vi "fpga_96ch-Main_dead_pixels.vi"   [LabVIEW 2011]
uses:
  <vilib>/Platform/TimedLoop/XDataNode/timing_clust.ctl
  <vilib>/Platform/TimedLoop/XDataNode/nitl_modes.ctl
  <vilib>/Platform/TimedLoop/XDataNode/wakeup.ctl
  <vilib>/Platform/TimedLoop/XDataNode/XDataNode.xnode
  <vilib>/Platform/TimedLoop/XDataNode/XDNodeRunTimeDep.lvlib
types:
  T1 = typedef "XDNodeRunTimeDep.lvlib/timing_clust.ctl" = cluster{"Expected End [f-1]":u64, "Actual End [f-1]":u64, "Finished Late? [f-1]":bool, "Expected End [i-1]":u64, "Actual End [i-1]":u64, "Finished Late? [i-1]":bool, "Expected Start [i]":u64, "Actual Start [i]":u64, "Expected Start [f]":u64, "Actual Start [f]":u64, "Source Name":string, "Structure Name":string, "Period":i64, "Deadline":i64, "Offset":i64, "Start":i64, "Priority":i32, "Timeout":i32, "Mode":T2, "Wakeup Reason":T3, "Error":errorcluster, "Source Type":string, "Secondary Source Type":string, "Global End Time":u64, "Global Start Time":u64, "Frame Duration":u64, "Iteration Duration":u64, "Assigned CPU":i32, "I/O Scan Engine Mode":u32}
  T2 = typedef "XDNodeRunTimeDep.lvlib/nitl_modes.ctl" = enum32{"No Change", "Process missed periods, maintain original phase", "Discard missed periods, maintain original phase", "Process missed periods, ignore original phase", "Discard missed periods, ignore original phase"}
  T3 = typedef "XDNodeRunTimeDep.lvlib/wakeup.ctl" = enum32{"Normal", "Aborted", "Asynchronous wakeup", "Timing source error", "Timed loop error", "Timeout"}
  T4 = cluster{"Connector0/DIO0":bool, "Connector0/DIO1":bool, "Connector0/DIO2":bool, "Connector0/DIO3":bool, "Connector0/DIO4":bool, "Connector0/DIO5":bool, "Connector0/DIO6":bool, "Connector0/DIO7":bool}
  T5 = cluster{"D0":bool, "D1":bool, "D2":bool, "D3":bool, "D4":bool, "D5":bool, "D6":bool, "D7":bool}
  T6 = cluster{"D0":u32, "D1 2":u32, "D2 3":u32, "D3 4":u32, "D4 5":u32, "D5 6":u32, "D6 7":u32, "D7 8":u32}
  T7 = typedef "Time Stamp Data.ctl" = cluster{"Timestamp":u32, "Data available":bool}
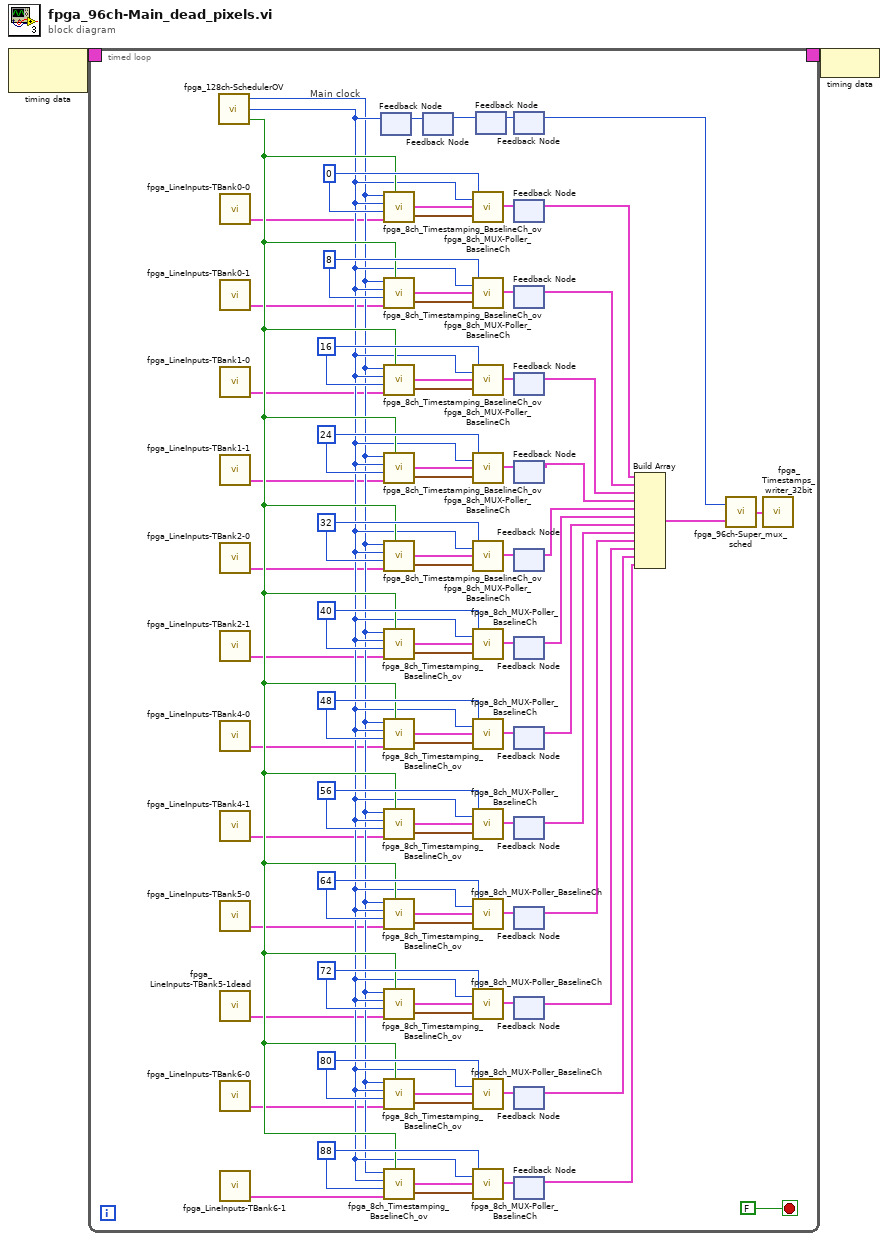
[diagram p0: block diagram]
diagram:
  n1 = node-c288() -> (w2:T1)  [unwired: 1 in]
  n2 = timed-loop {
    timing: w2 -> [_]
    timing-out: [_] -> w1
    stop <- FALSE stop-if-true
    w29 = u8 88 ("Baseline Ch")
    w33 = u8 80 ("Baseline Ch")
    w37 = u8 72 ("Baseline Ch")
    w41 = u8 64 ("Baseline Ch")
    w45 = u8 56 ("Baseline Ch")
    w49 = u8 48 ("Baseline Ch")
    w53 = u8 40 ("Baseline Ch")
    w57 = u8 32 ("Baseline Ch")
    w61 = u8 24 ("Baseline Ch")
    w65 = u8 16 ("Baseline Ch")
    w70 = u8 8 ("Baseline Ch")
    w81 = u8 0 ("Baseline Ch")
    # "Main clock"
    n3 = call "fpga_128ch-SchedulerOV.vi"() -> ("overflow"=w27:bool, "FIFO Schedule"=w26:u8, "Main clock"=w25:u32)  [unwired: 3 in]
    n4 = call "fpga_LineInputs-TBank0-0.vi"() -> ("DataLines"=w3:T4)  [unwired: 5 in]
    n5 = call "fpga_LineInputs-TBank0-1.vi"() -> ("DataLines"=w4:T4)  [unwired: 5 in]
    n6 = call "fpga_LineInputs-TBank1-0.vi"() -> ("DataLines"=w5:T4)  [unwired: 5 in]
    n7 = call "fpga_LineInputs-TBank1-1.vi"() -> ("DataLines"=w6:T4)  [unwired: 5 in]
    n8 = call "fpga_LineInputs-TBank2-0.vi"() -> ("DataLines"=w7:T4)  [unwired: 5 in]
    n9 = call "fpga_LineInputs-TBank2-1.vi"() -> ("DataLines"=w8:T4)  [unwired: 5 in]
    n10 = call "fpga_LineInputs-TBank4-0.vi"() -> ("DataLines"=w9:T4)  [unwired: 5 in]
    n11 = call "fpga_LineInputs-TBank4-1.vi"() -> ("DataLines"=w10:T4)  [unwired: 5 in]
    n12 = call "fpga_LineInputs-TBank5-0.vi"() -> ("DataLines"=w11:T4)  [unwired: 5 in]
    n13 = call "fpga_LineInputs-TBank5-1dead.vi"() -> ("DataLines"=w12:T4)  [unwired: 5 in]
    n14 = call "fpga_LineInputs-TBank6-0.vi"() -> ("DataLines"=w13:T4)  [unwired: 5 in]
    n15 = call "fpga_LineInputs-TBank6-1.vi"() -> ("DataLines"=w14:T4)  [unwired: 5 in]
    n16 = feedback #1() -> (w76:u8)  [unwired: 1 in]
    n17 = feedback-in #1(w26) -> ()
    n18 = call "fpga_8ch_Timestamping_BaselineCh_ov.vi"("Main clock"=w25, "Scheduler"=w26, "Baseline Ch"=w81, "Signal IN"=w3, "overflow"=w27) -> ("Data available"=w82:T5, "Timestamp bundle"=w83:T6)
    n19 = call "fpga_8ch_Timestamping_BaselineCh_ov.vi"("Main clock"=w25, "Scheduler"=w26, "Baseline Ch"=w70, "Signal IN"=w4, "overflow"=w27) -> ("Data available"=w71:T5, "Timestamp bundle"=w72:T6)
    n20 = call "fpga_8ch_Timestamping_BaselineCh_ov.vi"("Main clock"=w25, "Scheduler"=w26, "Baseline Ch"=w65, "Signal IN"=w5, "overflow"=w27) -> ("Data available"=w66:T5, "Timestamp bundle"=w67:T6)
    n21 = call "fpga_8ch_Timestamping_BaselineCh_ov.vi"("Main clock"=w25, "Scheduler"=w26, "Baseline Ch"=w61, "Signal IN"=w6, "overflow"=w27) -> ("Data available"=w62:T5, "Timestamp bundle"=w63:T6)
    n22 = call "fpga_8ch_Timestamping_BaselineCh_ov.vi"("Main clock"=w25, "Scheduler"=w26, "Baseline Ch"=w57, "Signal IN"=w7, "overflow"=w27) -> ("Data available"=w58:T5, "Timestamp bundle"=w59:T6)
    n23 = call "fpga_8ch_Timestamping_BaselineCh_ov.vi"("Main clock"=w25, "Scheduler"=w26, "Baseline Ch"=w53, "Signal IN"=w8, "overflow"=w27) -> ("Data available"=w54:T5, "Timestamp bundle"=w55:T6)
    n24 = call "fpga_8ch_Timestamping_BaselineCh_ov.vi"("Main clock"=w25, "Scheduler"=w26, "Baseline Ch"=w49, "Signal IN"=w9, "overflow"=w27) -> ("Data available"=w50:T5, "Timestamp bundle"=w51:T6)
    n25 = call "fpga_8ch_Timestamping_BaselineCh_ov.vi"("Main clock"=w25, "Scheduler"=w26, "Baseline Ch"=w45, "Signal IN"=w10, "overflow"=w27) -> ("Data available"=w46:T5, "Timestamp bundle"=w47:T6)
    n26 = call "fpga_8ch_Timestamping_BaselineCh_ov.vi"("Main clock"=w25, "Scheduler"=w26, "Baseline Ch"=w41, "Signal IN"=w11, "overflow"=w27) -> ("Data available"=w42:T5, "Timestamp bundle"=w43:T6)
    n27 = call "fpga_8ch_Timestamping_BaselineCh_ov.vi"("Main clock"=w25, "Scheduler"=w26, "Baseline Ch"=w37, "Signal IN"=w12, "overflow"=w27) -> ("Data available"=w38:T5, "Timestamp bundle"=w39:T6)
    n28 = call "fpga_8ch_Timestamping_BaselineCh_ov.vi"("Main clock"=w25, "Scheduler"=w26, "Baseline Ch"=w33, "Signal IN"=w13, "overflow"=w27) -> ("Data available"=w34:T5, "Timestamp bundle"=w35:T6)
    n29 = call "fpga_8ch_Timestamping_BaselineCh_ov.vi"("Main clock"=w25, "Scheduler"=w26, "Baseline Ch"=w29, "Signal IN"=w14, "overflow"=w27) -> ("Data available"=w30:T5, "Timestamp bundle"=w31:T6)
    n30 = feedback #2() -> (w75:u8)  [unwired: 1 in]
    n31 = feedback-in #2(w76) -> ()
    n32 = call "fpga_8ch_MUX-Poller_BaselineCh.vi"("Timestamp bundle"=w83, "Data available"=w82, "Scheduler"=w26, "Baseline CH"=w81) -> ("8Ch Timestamps"=w77:T7)
    n33 = call "fpga_8ch_MUX-Poller_BaselineCh.vi"("Timestamp bundle"=w72, "Data available"=w71, "Scheduler"=w26, "Baseline CH"=w70) -> ("8Ch Timestamps"=w69:T7)
    n34 = call "fpga_8ch_MUX-Poller_BaselineCh.vi"("Timestamp bundle"=w67, "Data available"=w66, "Scheduler"=w26, "Baseline CH"=w65) -> ("8Ch Timestamps"=w64:T7)
    n35 = call "fpga_8ch_MUX-Poller_BaselineCh.vi"("Timestamp bundle"=w63, "Data available"=w62, "Scheduler"=w26, "Baseline CH"=w61) -> ("8Ch Timestamps"=w60:T7)
    n36 = call "fpga_8ch_MUX-Poller_BaselineCh.vi"("Timestamp bundle"=w59, "Data available"=w58, "Scheduler"=w26, "Baseline CH"=w57) -> ("8Ch Timestamps"=w56:T7)
    n37 = call "fpga_8ch_MUX-Poller_BaselineCh.vi"("Timestamp bundle"=w55, "Data available"=w54, "Scheduler"=w26, "Baseline CH"=w53) -> ("8Ch Timestamps"=w52:T7)
    n38 = call "fpga_8ch_MUX-Poller_BaselineCh.vi"("Timestamp bundle"=w51, "Data available"=w50, "Scheduler"=w26, "Baseline CH"=w49) -> ("8Ch Timestamps"=w48:T7)
    n39 = call "fpga_8ch_MUX-Poller_BaselineCh.vi"("Timestamp bundle"=w47, "Data available"=w46, "Scheduler"=w26, "Baseline CH"=w45) -> ("8Ch Timestamps"=w44:T7)
    n40 = call "fpga_8ch_MUX-Poller_BaselineCh.vi"("Timestamp bundle"=w43, "Data available"=w42, "Scheduler"=w26, "Baseline CH"=w41) -> ("8Ch Timestamps"=w40:T7)
    n41 = call "fpga_8ch_MUX-Poller_BaselineCh.vi"("Timestamp bundle"=w39, "Data available"=w38, "Scheduler"=w26, "Baseline CH"=w37) -> ("8Ch Timestamps"=w36:T7)
    n42 = call "fpga_8ch_MUX-Poller_BaselineCh.vi"("Timestamp bundle"=w35, "Data available"=w34, "Scheduler"=w26, "Baseline CH"=w33) -> ("8Ch Timestamps"=w32:T7)
    n43 = call "fpga_8ch_MUX-Poller_BaselineCh.vi"("Timestamp bundle"=w31, "Data available"=w30, "Scheduler"=w26, "Baseline CH"=w29) -> ("8Ch Timestamps"=w28:T7)
    n44 = feedback #3() -> (w74:u8)  [unwired: 1 in]
    n45 = feedback-in #3(w75) -> ()
    n46 = feedback-in #4(w74) -> ()
    n47 = feedback #4() -> (w73:u8)  [unwired: 1 in]
    n48 = feedback-in #5(w77) -> ()
    n49 = feedback #5() -> (w78:T7)  [unwired: 1 in]
    n50 = feedback #6() -> (w68:T7)  [unwired: 1 in]
    n51 = feedback-in #6(w69) -> ()
    n52 = feedback #7() -> (w24:T7)  [unwired: 1 in]
    n53 = feedback-in #7(w64) -> ()
    n54 = feedback #8() -> (w23:T7)  [unwired: 1 in]
    n55 = feedback-in #8(w60) -> ()
    n56 = feedback #9() -> (w22:T7)  [unwired: 1 in]
    n57 = feedback-in #9(w56) -> ()
    n58 = feedback #10() -> (w21:T7)  [unwired: 1 in]
    n59 = feedback-in #10(w52) -> ()
    n60 = feedback #11() -> (w20:T7)  [unwired: 1 in]
    n61 = feedback-in #11(w48) -> ()
    n62 = feedback #12() -> (w19:T7)  [unwired: 1 in]
    n63 = feedback-in #12(w44) -> ()
    n64 = feedback #13() -> (w18:T7)  [unwired: 1 in]
    n65 = feedback-in #13(w40) -> ()
    n66 = feedback #14() -> (w17:T7)  [unwired: 1 in]
    n67 = feedback-in #14(w36) -> ()
    n68 = feedback #15() -> (w16:T7)  [unwired: 1 in]
    n69 = feedback-in #15(w32) -> ()
    n70 = feedback #16() -> (w15:T7)  [unwired: 1 in]
    n71 = feedback-in #16(w28) -> ()
    n72 = Build Array(w78, w68, w24, w23, w22, w21, w20, w19, w18, w17, w16, w15) -> (w80:T7[])
    n73 = call "fpga_96ch-Super_mux_sched.vi"("12 8Ch-timestamp-data array"=w80, "Scheduler"=w73) -> ("All Ch Timestamps"=w79:T7)
    n74 = call "fpga_Timestamps_writer_32bit.vi"("All Ch Timestamps"=w79) -> ()  [unwired: 1 in]
  }
  n75 = node-c288(w1) -> ()
